vi "ReadPropertyInfo.vi"(7 "physical channel":string="Scratchpad64/NI.Scratchpad.AsDouble.PolynomialThermocouple", 8 "error in (no error)":errorcluster, 10 "Caps":T1, 11 "property":string="Scratchpad64/NI.Scratchpad.AsDouble.PolynomialThermocouple") -> (0 "error out":errorcluster, 3 "property info":T10)   [LabVIEW 2017]
uses:
  Ctrl/Property.ctl
  Ctrl/Bitfield.ctl
  Ctrl/Register.ctl
  Ctrl/ScaleType.ctl
  Ctrl/Scale.ctl
  Ctrl/EnumValue.ctl
  Ctrl/Enum.ctl
  Ctrl/PhysicalChannel.ctl
  Ctrl/Caps.ctl
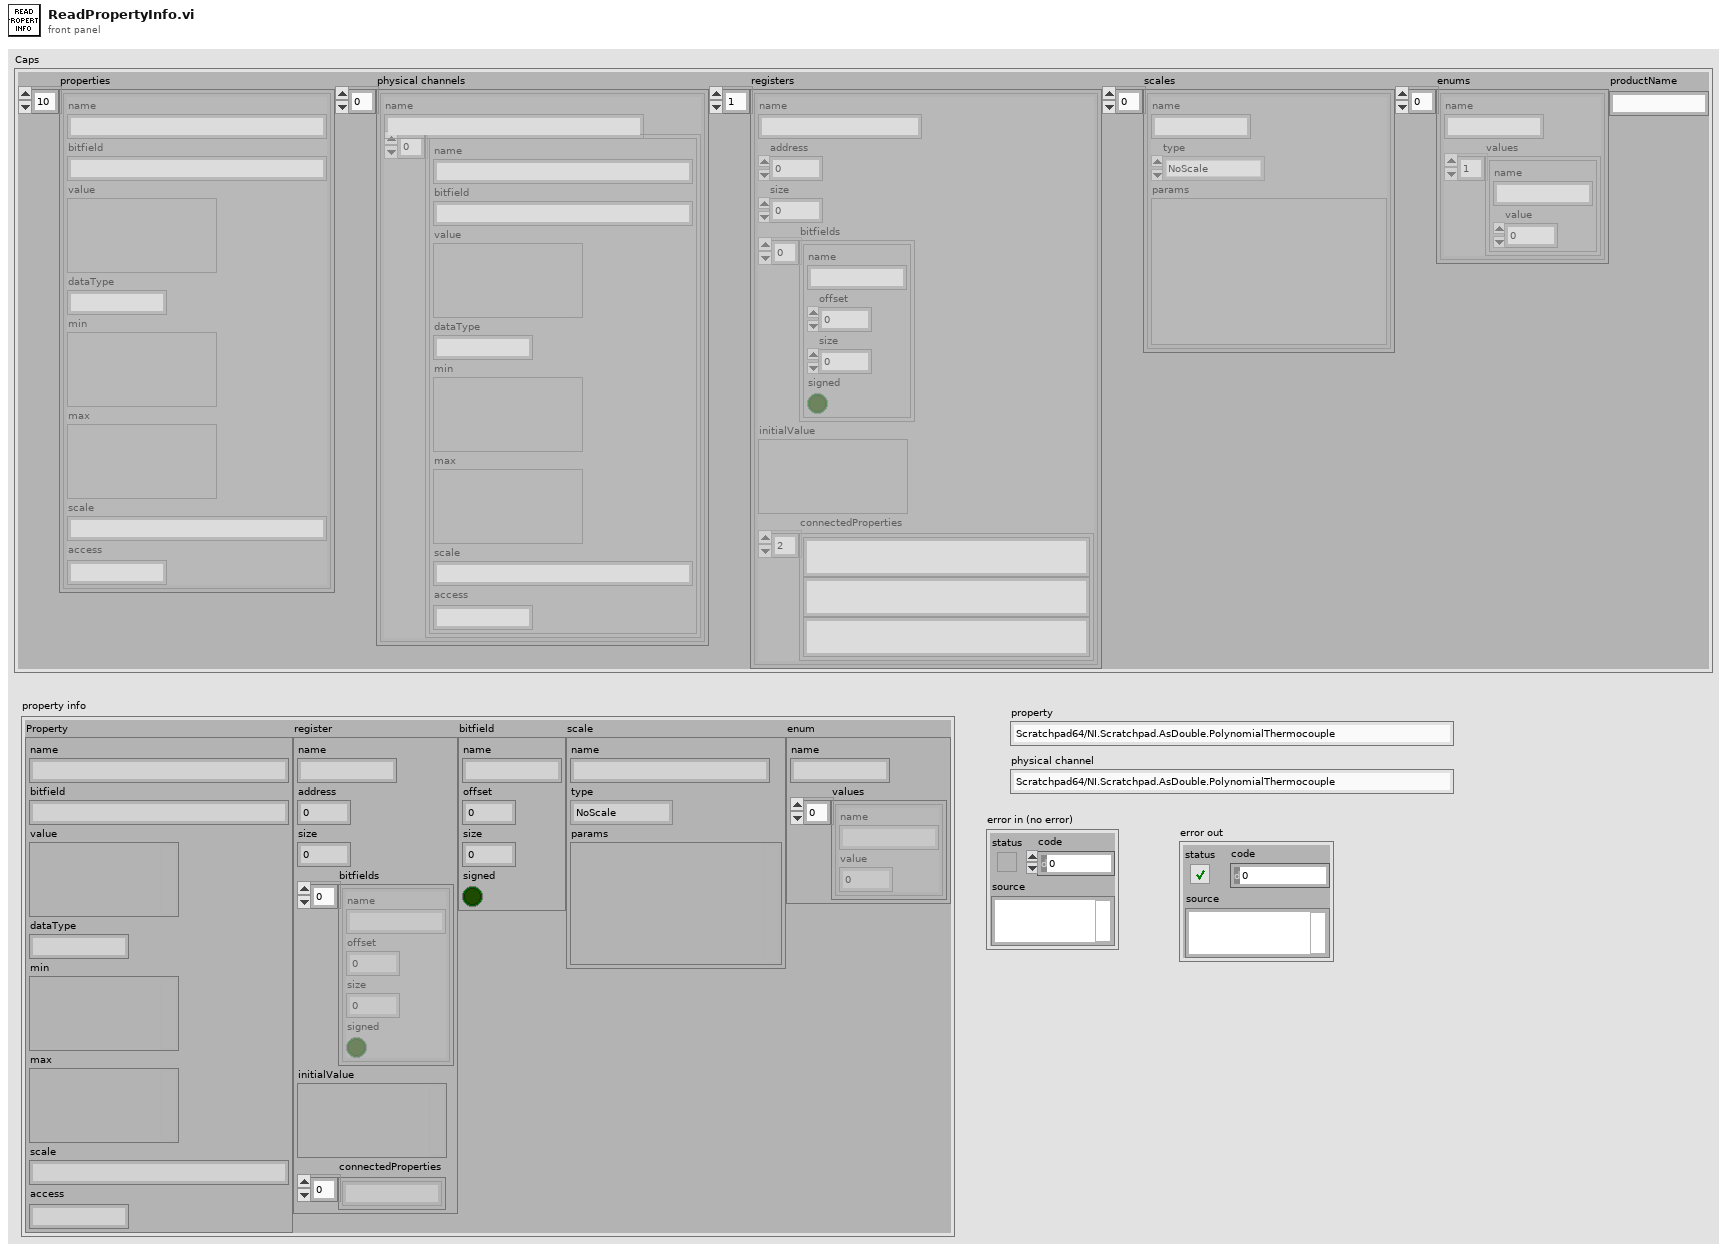
[diagram p1: front panel]
types:
  T1 = typedef "Caps.ctl" = cluster{"properties":T2[], "physical channels":T3[], "registers":T4[], "scales":T6[], "enums":T8[], "productName":string}
  T2 = typedef "Property.ctl" = cluster{"name":string, "bitfield":string, "value":variant, "dataType":string, "min":variant, "max":variant, "scale":string, "access":string}
  T3 = typedef "PhysicalChannel.ctl" = cluster{"name":string, "properties":T2[]}
  T4 = typedef "Register.ctl" = cluster{"name":string, "address":i32, "size":i32, "bitfields":T5[], "initialValue":variant, "connectedProperties":string[]}
  T5 = typedef "Bitfield.ctl" = cluster{"name":string, "offset":i32, "size":i32, "signed":bool}
  T6 = typedef "Scale.ctl" = cluster{"name":string, "type":T7, "params":variant}
  T7 = typedef "ScaleType.ctl" = enum16{"NoScale", "Table", "Polynomial", "Linear"}
  T8 = typedef "Enum.ctl" = cluster{"name":string, "values":T9[]}
  T9 = typedef "EnumValue.ctl" = cluster{"name":string, "value":i32}
  T10 = cluster{"Property":T2, "register":T4, "bitfield":T5, "scale":T6, "enum":T8}
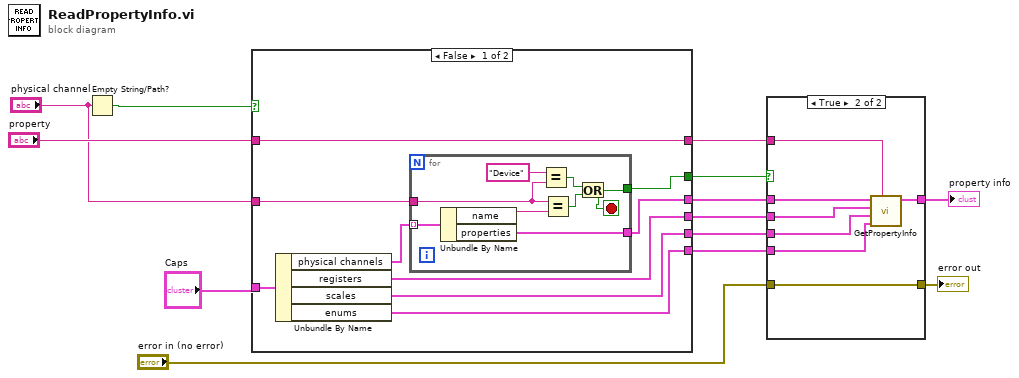
[diagram p0: block diagram]
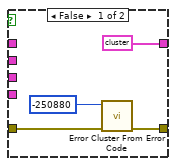
[diagram p2: hidden frame]
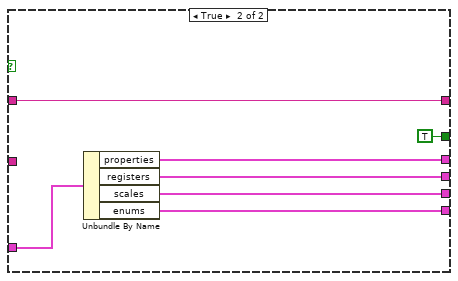
[diagram p3: hidden frame]
diagram:
  n1 = Empty String/Path?(string/path="physical channel") -> (empty?=w3:bool)
  n2 = case shown="False" w3 {
    tunnel: "Caps" -> [w22 w37]
    tunnel: [w15 w31] -> w9
    tunnel: [w20 w36] -> w13
    tunnel: [w19 w35] -> w12
    tunnel: [w18 w34] -> w11
    tunnel: [w17 w33] -> w10
    tunnel: [w16 TRUE] -> w6
    tunnel: "property" -> [w15 w31]
    tunnel: "physical channel" -> [w14 _]
    frame False {
      n3 = Unbundle By Name(w22) -> ("physical channels"=w21:T3[], "registers"=w19:T4[], "scales"=w18:T6[], "enums"=w17:T8[])
      n4 = for {
        tunnel: w21 -> [w29] mode=indexing
        tunnel: w14 -> [w27]
        tunnel: [w28] -> w20
        tunnel: [w23] -> w16
        stop <- w23 stop-if-true
        n5 = Unbundle By Name(w29) -> ("name"=w30:string, "properties"=w28:T2[])
        n6 = Equal?(x="Device", y=w27) -> (x = y?=w25:bool)
        n7 = Equal?(x=w27, y=w30) -> (x = y?=w24:bool)
        n8 = Or(x=w25, y=w24) -> (x .or. y?=w23:bool)
      }
    }
    frame True {
      n9 = Unbundle By Name(w37) -> ("properties"=w36:T2[], "registers"=w35:T4[], "scales"=w34:T6[], "enums"=w33:T8[])
    }
  }
  n10 = case shown="True" w6 {
    tunnel: w13 -> [_ w44]
    tunnel: w12 -> [_ w48]
    tunnel: w11 -> [_ w42]
    tunnel: w10 -> [_ w47]
    tunnel: w9 -> [_ w43]
    tunnel: [T10 {"Property"={"name"="", "bitfield"="", "value"=variant, "dataType"="", "min"=variant, "max"=variant, "scale"="", "access"=""}, "register"={"name"="", "address"=0, "size"=0, "bitfields"=[], "initialValue"=variant, "connectedProperties"=[]}, "bitfield"={"name"="", "offset"=0, "size"=0, "signed"=FALSE}, "scale"={"name"="", "type"=enum."NoScale", "params"=variant}, "enum"={"name"="", "values"=[]}} ("property info") w46] -> w8
    tunnel: "error in (no error)" -> [w40 w45]
    tunnel: [w39 w45] -> w4
    frame False {
      n11 = call <vilib>:"Error Cluster From Error Code.vi"("error in (no error)"=w40, "error code (0)"=-250880) -> ("error out"=w39:errorcluster)  [unwired: 7 in]
    }
    frame True {
      n12 = call "GetPropertyInfo.vi"("property"=w43, "enums"=w47, "scales"=w42, "registers"=w48, "properties"=w44) -> ("property info"=w46:T10)  [unwired: 6 in]
    }
  }
  "property info" <- w8
  "error out" <- w4
